vi "Template Delete.vi"(8 "error in (no error)":errorcluster, 10 "Template Record":T1, 11 "Connection Refnum":T2) -> (0 "error out":errorcluster, 3 "Connection Refnum":T2)   [LabVIEW 2011]
uses:
  Summitek EXT/ODBC/SQL Controls/Connection Refnum.ctl
  Template Record.ctl
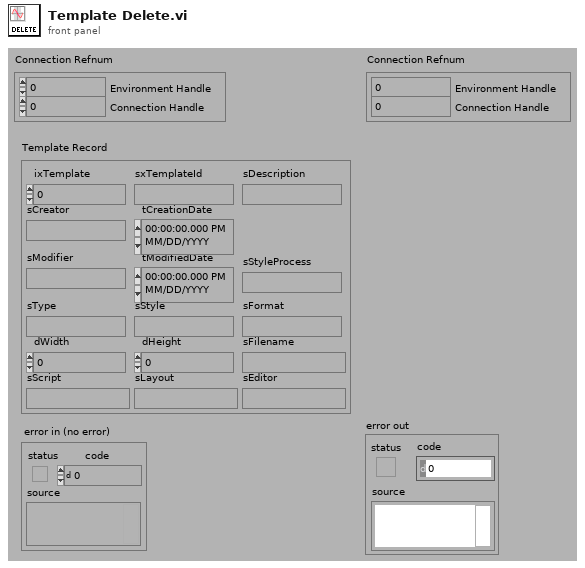
[diagram p1: front panel]
types:
  T1 = typedef "Template Record.ctl" = cluster{"ixTemplate":i32, "sxTemplateId":string, "sDescription":string, "sCreator":string, "tCreationDate":timestamp, "sModifier":string, "tModifiedDate":timestamp, "sType":string, "sStyle":string, "sFormat":string, "dWidth":dbl, "dHeight":dbl, "sFilename":string, "sScript":string, "sLayout":string, "sEditor":string, "sStyleProcess":string}
  T2 = typedef "Connection Refnum.ctl" = cluster{"Environment Handle":i32, "Connection Handle":i32}
  T3 = typedef "Statement Refnum.ctl" = cluster{"Statement Handle":i32, "Parameter Number":u16}
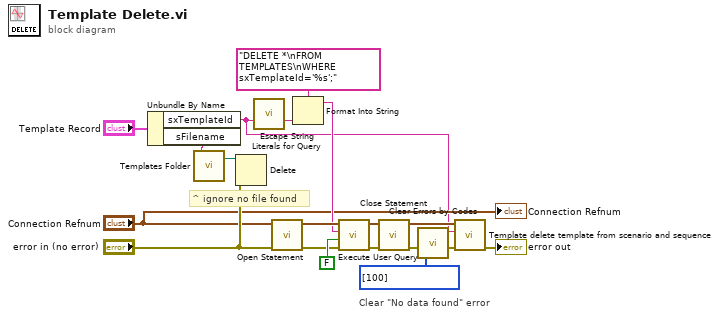
[diagram p0: block diagram]
diagram:
  # "^ ignore no file found"
  # "Clear \"No data found\" error"
  n1 = Unbundle By Name("Template Record") -> ("sxTemplateId"=w1:string, "sFilename"=w5:string)
  n2 = call "Templates Folder.vi"("Relative Path (\"\")"=w5) -> ("Templates Folder"=w8:path)  [unwired: 2 out]
  n3 = Delete(path (use dialog)=w8, error in="error in (no error)") -> ()  [unwired: 6 out]
  n4 = call "Escape String Literals for Query.vi"("String"=w1) -> ("escaped String"=w7:string)  [unwired: 1 in, 13 out]
  n5 = call "Open Statement.vi"("error in (no error)"="error in (no error)", "Connection Refnum"="Connection Refnum") -> ("error out"=w15:errorcluster, "Statement Refnum"=w14:T3)  [unwired: 4 out]
  n6 = Format Into String(format string="DELETE *\nFROM TEMPLATES\nWHERE sxTemplateId='%s';" ("User Query"), w7) -> (resulting string=w13:string)  [unwired: 2 in, 1 out]
  n7 = call "Execute User Query.vi"("error in (no error)"=w15, "Return Data? (f)"=FALSE, "User Query"=w13, "Statement Refnum"=w14) -> ("error out"=w16:errorcluster, "Statement Refnum"=w17:T3)  [unwired: 2 out]
  n8 = call "Close Statement.vi"("error in (no error)"=w16, "Statement Refnum"=w17) -> ("error out"=w11:errorcluster)  [unwired: 5 out]
  n9 = call "Clear Errors by Codes.vi"("Error Codes\nto Clear (Empty)"=i32[] [100] ("Error Codes\nto Clear (Empty)"), "error in (no error)"=w11) -> ("error out"=w4:errorcluster)  [unwired: 5 out]
  n10 = call "Template delete template from scenario and sequence.vi"("error in (no error)"=w4, "deleted template name"=w1, "Connection Refnum"="Connection Refnum") -> ("error out"=→"error out":errorcluster)  [unwired: 8 out]
  "Connection Refnum" <- "Connection Refnum"
